vi "SRV_Get Enum Info (Variant Input).vi"(6 "Variant (Enum)":variant) -> (0 "Enum Strings":string[](array[string]), 2 "Enum Size":i32, 3 "Enum Name":string)   [LabVIEW 2014]
doc: "Returns information about an enumerated type. Wire any Enum to the Variant (Enum) input.\n\n\n<B>Note:</B> Type string code values might change in future LabVIEW versions. This version of the VI works for:\nLabVIEW 5.1.1, LabVIEW 6.0.2, LabVIEW 7.x, LabVIEW 8.x, LabVIEW 9.x (moving from 'Flatten to String' to 'Variant to Flattened String')\n\n<B>Keywords:</B> enum, enumerated type\n\n<B>Initial Developer:</B> Mike Schultz"
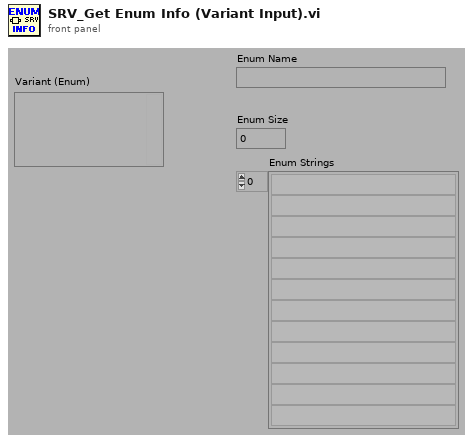
[diagram p1: front panel]
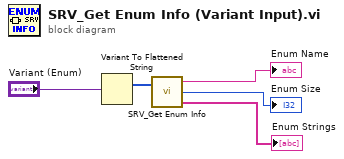
[diagram p0: block diagram]
diagram:
  n1 = Variant To Flattened String(Variant="Variant (Enum)") -> (1:w5:i16[])  [unwired: 1 out]
  n2 = call "SRV_Get Enum Info.vi"("Enum type string"=w5) -> ("Enum Strings"=→"Enum Strings":string[], "Enum Size"=→"Enum Size":i32, "Enum Name"=→"Enum Name":string)  [unwired: 3 in]
